vi "WhiteNoiseToTXTFile.vi"(8 "Gain":dbl=3.0, 9 "Filter":bool=TRUE, 10 "Save":bool, 11 "Generate New Data":bool) -> (0 "error out":errorcluster, 3 "output waveform":waveform(dbl))   [LabVIEW 2022 SP3]
uses:
  <vilib>/Analysis/3filter.llb/Filter Passband Type.ctl
  <vilib>/Analysis/3filter.llb/Butterworth Filter (DBL).vi
  <vilib>/measure/maspectr.llb/FFT Spectrum (Mag-Phase) for 1 Chan.vi
  <vilib>/measure/maspectr.llb/FFT Power Spectrum and PSD for 1 Chan.vi
  <vilib>/Waveform/WDTFileIO.llb/Write Waveform to File.vi
  <vilib>/Waveform/WDTFileIO.llb/Read Waveform from File.vi
  <vilib>/measure/NI_MABase.lvlib
  <vilib>/measure/NI_MAPro.lvlib
  <vilib>/Analysis/NI_AALBase.lvlib
panel:
  in  "error in (no error)":errorcluster
  out "Filtered PSD":cluster{"f0":dbl, "df":dbl, "magnitude":dbl[]}(graph)
  out "Filtered FFT":cluster{"f0":dbl, "df":dbl, "magnitude":dbl[]}(graph)
  out "FFT":cluster{"f0":dbl, "df":dbl, "magnitude":dbl[]}(graph)
  out "PSD":cluster{"f0":dbl, "df":dbl, "magnitude":dbl[]}(graph)
  out "Waveform Chart":waveform(dbl)(graph)
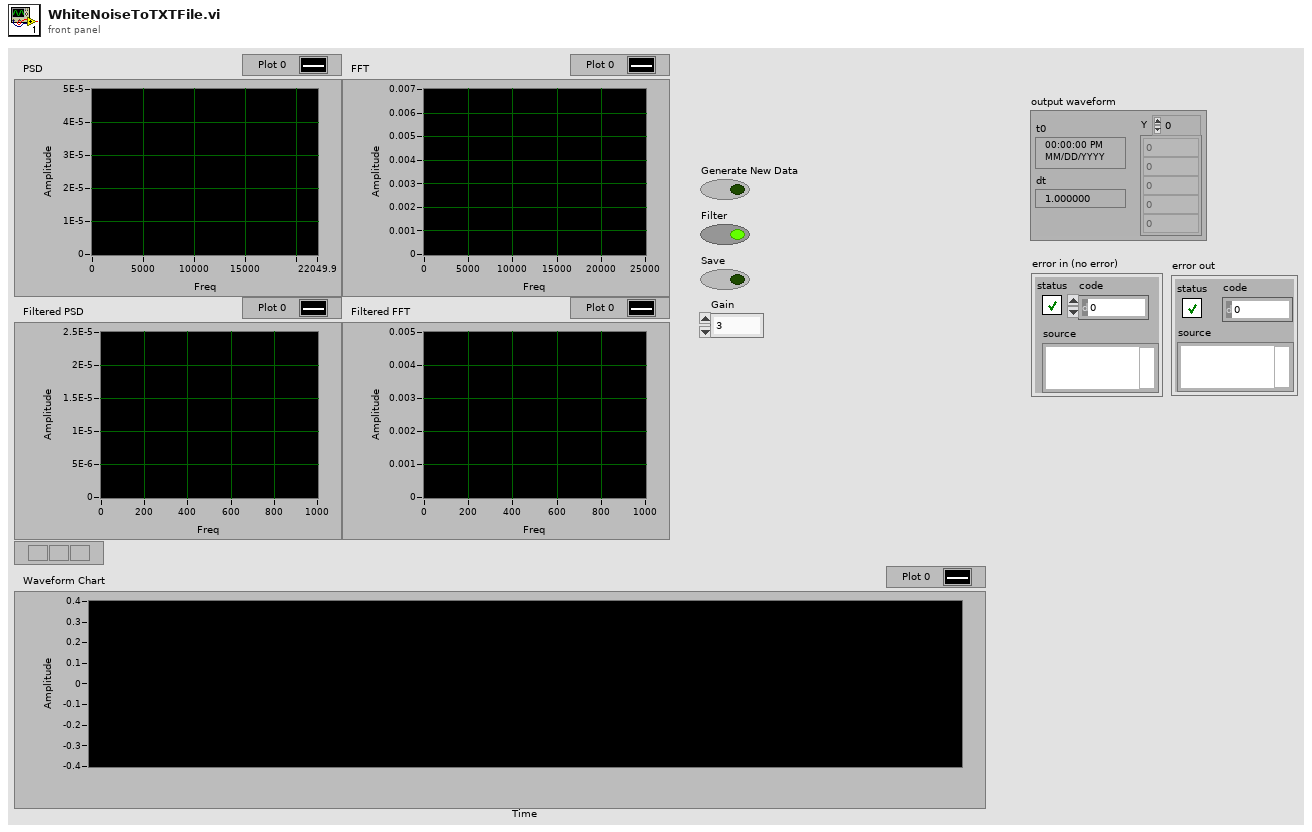
[diagram p1: front panel]
types:
  T1 = typedef "NI_AALBase.lvlib/Filter Passband Type.ctl" = enum32{"Lowpass", "Highpass", "Bandpass", "Bandstop"}
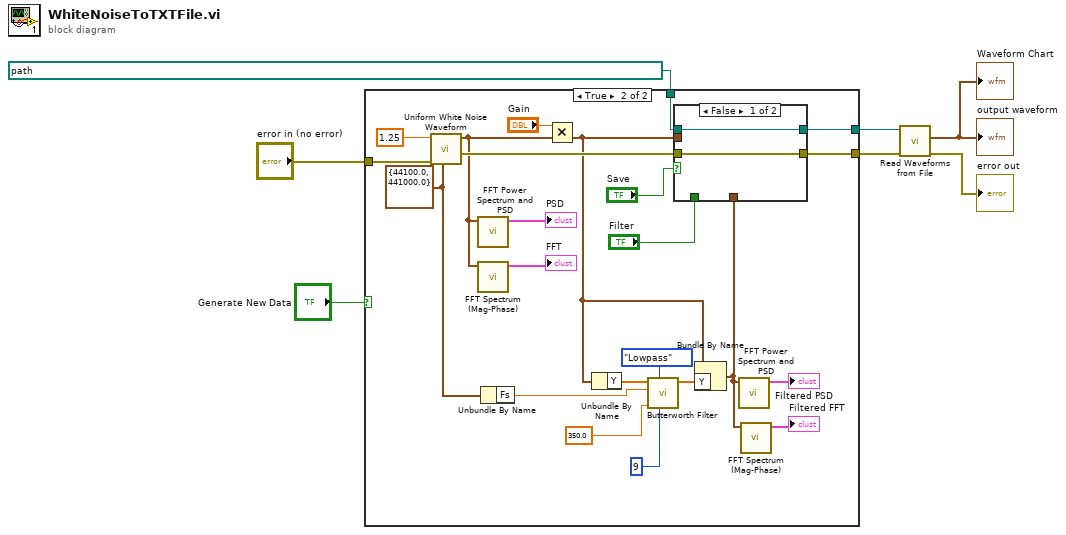
[diagram p0: block diagram]
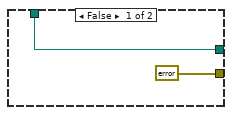
[diagram p2: hidden frame]
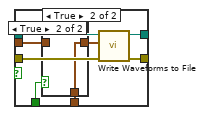
[diagram p3: hidden frame]
diagram:
  n1 = case shown="True" "Generate New Data" {
    tunnel: path "C:/Users/LAV-UFSC-2023/Documents/LAV-TCC/Dados-Experimentos/ExperimentosApresentação/standard_excitation.txt" ("file path (dialog if empty)") -> [w8 w32]
    tunnel: [errorcluster {"status"=FALSE, "code"=0, "source"=""} ("error out") w31] -> w6
    tunnel: [w8 w30] -> w5
    tunnel: "error in (no error)" -> [_ w12]
    frame False {
    }
    frame True {
      w22 = cluster{"Fs":dbl, "#s":dbl} {"Fs"=44100.0, "#s"=441000.0} ("sampling info")
      n2 = call <vilib>:"Uniform White Noise Waveform.vi"("sampling info"=w22, "error in (no error)"=w12, "amplitude"=1.25 ("standard deviation")) -> ("error out"=w28:errorcluster, "signal out"=w16:waveform(dbl))  [unwired: 7 in]
      n3 = call-poly <vilib>:"FFT Power Spectrum and PSD.vi"("time signal"=w16) -> ("Power Spectrum / PSD"=→"PSD":cluster{"f0":dbl, "df":dbl, "magnitude":dbl[]})  [unwired: 7 in, 3 out]
      n4 = call-poly <vilib>:"FFT Spectrum (Mag-Phase).vi"("time signal"=w16) -> ("magnitude"=→"FFT":cluster{"f0":dbl, "df":dbl, "magnitude":dbl[]})  [unwired: 6 in, 4 out]
      n5 = Unbundle By Name(w22) -> ("Fs"=w21:dbl)
      n6 = Multiply(x="Gain", y=w16) -> (x*y=w11:waveform(dbl))
      n7 = Unbundle By Name(w11) -> ("Y"=w23:dbl[])
      n8 = call-poly <vilib>:"Butterworth Filter.vi"("order"=9, "filter type"=Filter_Passband_Type."Lowpass", "low cutoff freq: fl"=350.0 ("high cutoff freq: fh"), "sampling freq: fs"=w21, "X"=w23) -> ("Filtered X"=w15:dbl[])  [unwired: 3 in, 1 out]
      n9 = Bundle By Name(cluster=w11, "Y"=w15) -> (w13:waveform(dbl))
      n10 = case shown="False" "Save" {
        tunnel: w32 -> [w34 w42]
        tunnel: w28 -> [w33 w41]
        tunnel: [w33 w40] -> w31
        tunnel: [w34 w39] -> w30
        tunnel: w11 -> [_ w37]
        tunnel: "Filter" -> [_ w38]
        tunnel: w13 -> [_ w35]
        frame False {
        }
        frame True {
          n11 = case shown="True" w38 {
            tunnel: w37 -> [w43 _]
            tunnel: [w43 w44] -> w36
            tunnel: w35 -> [_ w44]
            frame False {
            }
            frame True {
            }
          }
          n12 = call-poly <vilib>:"Write Waveforms to File.vi"("error in (no error)"=w41, "waveform"=w36, "file path (dialog if empty)"=w42) -> ("error out"=w40:errorcluster, "new file path (Not A Path if cancelled)"=w39:path)  [unwired: 7 in]
        }
      }
      n13 = call-poly <vilib>:"FFT Power Spectrum and PSD.vi"("time signal"=w13) -> ("Power Spectrum / PSD"=→"Filtered PSD":cluster{"f0":dbl, "df":dbl, "magnitude":dbl[]})  [unwired: 7 in, 3 out]
      n14 = call-poly <vilib>:"FFT Spectrum (Mag-Phase).vi"("time signal"=w13) -> ("magnitude"=→"Filtered FFT":cluster{"f0":dbl, "df":dbl, "magnitude":dbl[]})  [unwired: 6 in, 4 out]
    }
  }
  n15 = call-poly <vilib>:"Read Waveforms from File.vi"("error in (no error)"=w6, "file path (dialog if empty)"=w5) -> ("error out"=→"error out":errorcluster, "first waveform in record"=→"Waveform Chart" →"output waveform":waveform(dbl))  [unwired: 4 in, 2 out]
